vi "Mass Measurement.vi"(4 "error in (no error)":errorcluster, 5 "Mass":i8=1 min=1 max=100 step=1, 6 "Timeout Limit":dbl format="%.2f", 7 "VISA Resource Name":refnum<visa-resource-name>="ASRL1::INSTR") -> (0 "error out":errorcluster, 1 "Timeout":bool, 2 "Partial Pressure Sensitivity Factor":string, 3 "Partial Pressure (torr)":dbl[](graph))   [LabVIEW 2019]
uses:
  Serial Support VISA.llb/Serial Actions.ctl
panel:
  in  "Delay (s)":dbl format="%.2f"
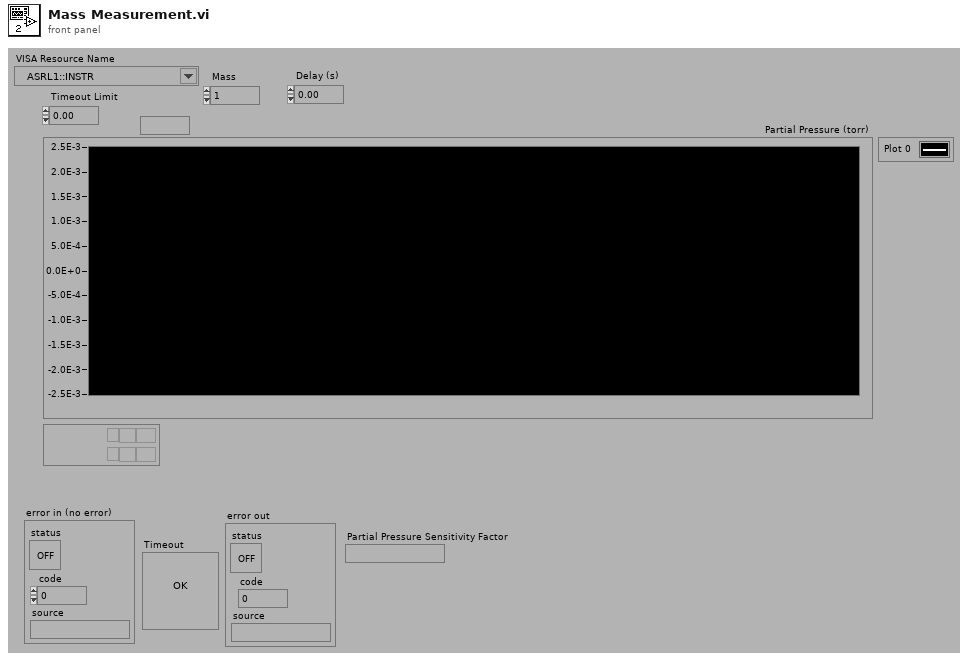
[diagram p1: front panel]
types:
  T1 = typedef "Serial Actions.ctl" = enum16{"Init", "Break", "Clear Buffer", "Write", "Read", "N Bytes", "Lock", "Unlock", "Close"}
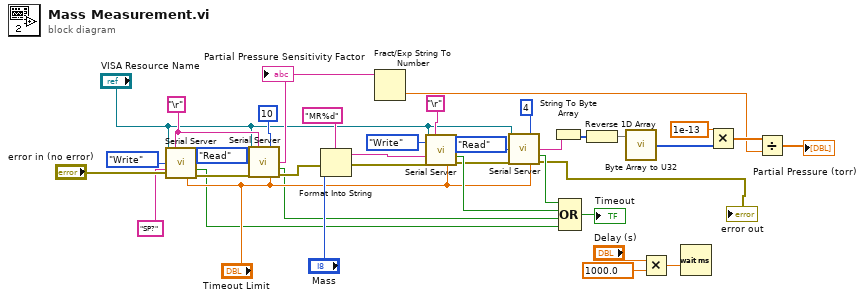
[diagram p0: block diagram]
diagram:
  w9 = "\r" ("EOT Chars (cr/lf)")
  n1 = call "Serial Server.vi"("VISA Resource Name"="VISA Resource Name", "EOT Chars (cr/lf)"=w9, "Action"=Serial_Actions."Write", "String To Send"="SP?", "error in (no error)"="error in (no error)", "Timeout Limit(sec)"="Timeout Limit") -> ("Timeout"=w10:bool, "error out"=w21:errorcluster)  [unwired: 5 in, 3 out]
  n2 = call "Serial Server.vi"("VISA Resource Name"="VISA Resource Name", "EOT Chars (cr/lf)"=w9, "Max Char to Read"=10, "Action"=Serial_Actions."Read", "error in (no error)"=w21, "Timeout Limit(sec)"="Timeout Limit") -> ("Serial Read"=w20:string, "Timeout"=w11:bool, "error out"=w18:errorcluster)  [unwired: 5 in, 2 out]
  "Partial Pressure Sensitivity Factor" <- w20
  n3 = Format Into String(format string="MR%d", error in=w18, "Mass") -> (resulting string=w30:string, error out=w29:errorcluster)  [unwired: 1 in]
  n4 = Fract/Exp String To Number(string=w20) -> (number=w13:dbl)  [unwired: 3 in, 1 out]
  n5 = call "Serial Server.vi"("VISA Resource Name"="VISA Resource Name", "EOT Chars (cr/lf)"="\r", "Action"=Serial_Actions."Write", "String To Send"=w30, "error in (no error)"=w29, "Timeout Limit(sec)"="Timeout Limit") -> ("Timeout"=w36:bool, "error out"=w34:errorcluster)  [unwired: 5 in, 3 out]
  n6 = call "Serial Server.vi"("VISA Resource Name"="VISA Resource Name", "Max Char to Read"=4, "Action"=Serial_Actions."Read", "error in (no error)"=w34, "Timeout Limit(sec)"="Timeout Limit") -> ("Serial Read"=w25:string, "Timeout"=w35:bool, "error out"=→"error out":errorcluster)  [unwired: 6 in, 2 out]
  n7 = String To Byte Array(string=w25) -> (unsigned byte array=w24:u8[])
  n8 = Compound Arithmetic op=OR(w35, w36, w11, w10) -> (→"Timeout":bool)
  n9 = Reverse 1D Array(array=w24) -> (reversed array=w4:u8[])
  n10 = call "Byte Array to U32.vi"("Input Bytes"=w4) -> ("Output Integers"=w23:i32[])
  n11 = Multiply(x="Delay (s)", y=1000.0) -> (x*y=w5:dbl)
  n12 = Wait (ms)(milliseconds to wait=w5) -> ()  [unwired: 1 out]
  n13 = Multiply(x=1e-13, y=w23) -> (x*y=w14:dbl[])
  n14 = Divide(x=w14, y=w13) -> (x/y=→"Partial Pressure (torr)":dbl[])
